vi "Enqueue Message.vi"(6 "Priority Message? (F)":bool, 8 "error in (no error)":errorcluster, 9 "Message Data":variant, 10 "Message":string, 11 "Process In":refnum<class "Process.lvclass">) -> (0 "error out":errorcluster, 3 "Process Out":refnum<class "Process.lvclass">)   [LabVIEW 2020, in "Process.lvclass"]
doc: "For a regular message, enqueue the message. For a priority message, enqueue it at the front of the queue."
uses:
  Process.lvclass
  Message Cluster.ctl
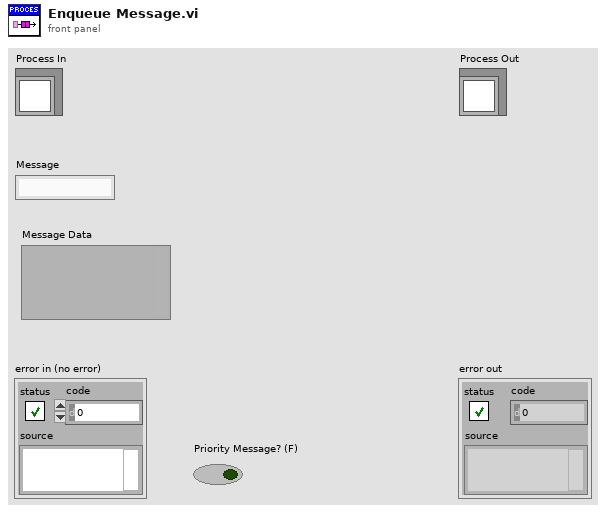
[diagram p1: front panel]
types:
  T1 = typedef "Process.lvclass/Message Cluster.ctl" = cluster{"Message":string, "Message Data":variant}
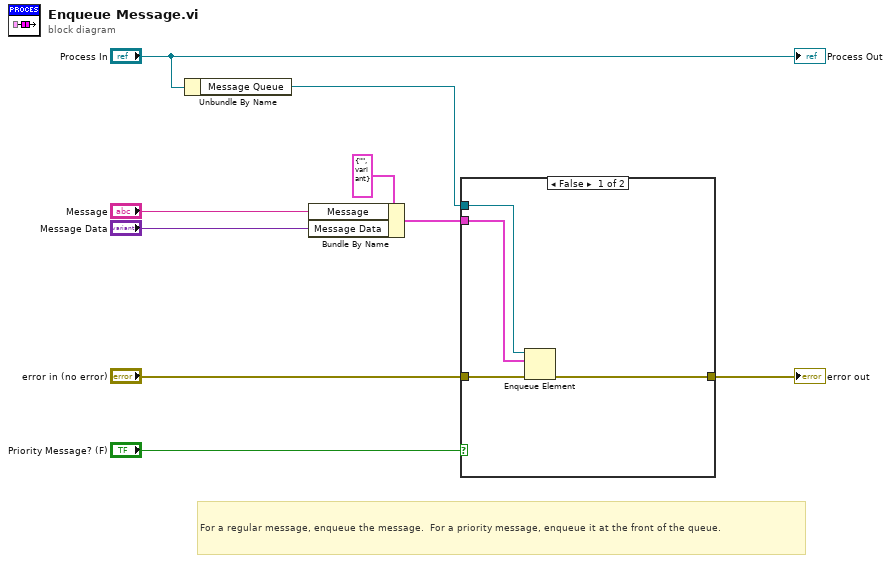
[diagram p0: block diagram]
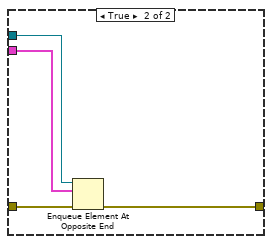
[diagram p2: hidden frame]
diagram:
  # "For a regular message, enqueue the message.  For a priority message, enqueue it at the front of the queue."
  n1 = Unbundle By Name("Process In") -> ("Message Queue"=w8:refnum<queue>)
  n2 = Bundle By Name(cluster=T1 {"Message"="", "Message Data"=variant} ("Message Cluster"), "Message"="Message", "Message Data"="Message Data") -> (w2:T1)
  n3 = case shown="False" "Priority Message? (F)" {
    tunnel: "error in (no error)" -> [w13 w17]
    tunnel: [w12 w16] -> w6
    tunnel: w8 -> [w11 w15]
    tunnel: w2 -> [w10 w14]
    frame False {
      n4 = Enqueue Element(queue=w11, element=w10, error in (no error)=w13) -> (error out=w12:errorcluster)  [unwired: 1 in, 2 out]
    }
    frame True {
      n5 = Enqueue Element At Opposite End(queue=w15, element=w14, error in (no error)=w17) -> (error out=w16:errorcluster)  [unwired: 1 in, 2 out]
    }
  }
  "error out" <- w6
  "Process Out" <- "Process In"
